vi "Test Lift Core.vi"(8 "Speed":dbl, 11 "Target Height":dbl) -> ()   [LabVIEW 2014]
uses:
  Begin/Global RefNums.vi
  Begin/Global Variables.vi
  <vilib>/addons/control/pid/pid.llb/PID (DBL).vi
  <vilib>/addons/control/pid/NI_PID_pid.lvlib
panel:
  in  "Clear Graph":bool
  out "Graph":cluster{"X":dbl, "Y":dbl}[](graph)
  in  "Speed Offset":dbl
  in  "Right PID gains":T1={"proportional gain (Kc)"=0.002, "integral time (Ti, min)"=0.0, "derivative time (Td, min)"=0.0005} {"derivative time (Td, min)" format="%.7f"; "integral time (Ti, min)" format="%.7f"; "proportional gain (Kc)" format="%.7f"}
  in  "Left PID gains":T1={"proportional gain (Kc)"=0.002, "integral time (Ti, min)"=0.0, "derivative time (Td, min)"=0.0005} {"derivative time (Td, min)" format="%.7f"; "integral time (Ti, min)" format="%.7f"; "proportional gain (Kc)" format="%.7f"}
  in  "Velocity gains":T1={"proportional gain (Kc)"=0.002, "integral time (Ti, min)"=0.0, "derivative time (Td, min)"=0.0} {"derivative time (Td, min)" format="%.7f"; "integral time (Ti, min)" format="%.7f"; "proportional gain (Kc)" format="%.7f"}
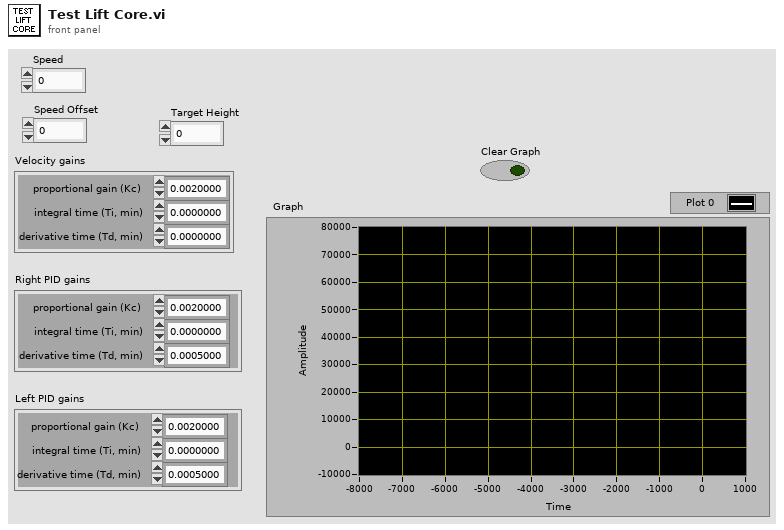
[diagram p1: front panel]
types:
  T1 = cluster{"proportional gain (Kc)":dbl, "integral time (Ti, min)":dbl, "derivative time (Td, min)":dbl}
  T2 = typedef "WPI_EncoderDevRef.ctl" = cluster{"DevStatus":errorcluster, "EncoderIndex":T3, "CounterIndex":T4, "DistancePerCount":dbl, "Decoding Type":T5}
  T3 = typedef "FPGA_EncoderIdx.ctl" = enum8{"Enc 0", "Enc 1", "Enc 2", "Enc 3", "Enc 4", "Enc 5", "Enc 6", "Enc 7", "Invalid"}
  T4 = typedef "FPGA_CounterCtrSystemIndex.ctl" = enum8{"Ctr 0", "Ctr 1", "Ctr 2", "Ctr 3", "Ctr 4", "Ctr 5", "Ctr 6", "Ctr 7", "Invalid"}
  T5 = typedef "WPI_EncoderType.ctl" = enum16{"1x", "2x", "4x"}
  T6 = typedef "WPI_MotorControlDeviceRef.ctl" = cluster{"DeviceStatus":errorcluster, "Type":T7, "PWM":cluster{"Controller":T8, "PWM Channel":T9, "DeadBand":T10}, "CAN":cluster{"Device Number":u8, "Control Mode":T11, "Semaphore":T12, "Max Vout":dbl, "TalonSRX Control Mode":T13}, "Invert":bool, "TransformRef":T14, "InvTransformRef":T14}
  T7 = typedef "WPI_MotorControlType.ctl" = enum16{"PWM", "CAN", "CANTalonSRX"}
  T8 = typedef "FPGA_TypedefDigitalModule.ctl" = enum16{"Controller 1"}
  T9 = typedef "FPGA_DIOPWMChannel.ctl" = enum8{"PWM 0", "PWM 1", "PWM 2", "PWM 3", "PWM 4", "PWM 5", "PWM 6", "PWM 7", "PWM 8", "PWM 9", "PWM MXP 0", "PWM MXP 1", "PWM MXP 2", "PWM MXP 3", "PWM MXP 4", "PWM MXP 5", "PWM MXP 6", "PWM MXP 7", "PWM MXP 8", "PWM MXP 9", "Invalid"}
  T10 = typedef "WPI_PWMDeadband.ctl" = cluster{"Name":string, "maxPositivePwm":i32, "minPositivePwm":i32, "centerPwm":i32, "maxNegativePwm":i32, "minNegativePwm":i32, "angularRange":u16}
  T11 = typedef "WPI_CANJaguar_ControlMode.ctl" = enum8{"Percent VBus", "Current", "Speed", "Position", "Voltage"}
  T12 = typedef "Semaphore RefNum" = refnum<k1>
  T13 = typedef "WPI_CANTalonSRX_APIControlMode.ctl" = enum8{"Percent VBus", "Speed", "Position", "Slave", "Unchanged / Invalid"}
  T14 = typedef "WPI_PWMTransform_ConPane.ctl" = refnum<vi>
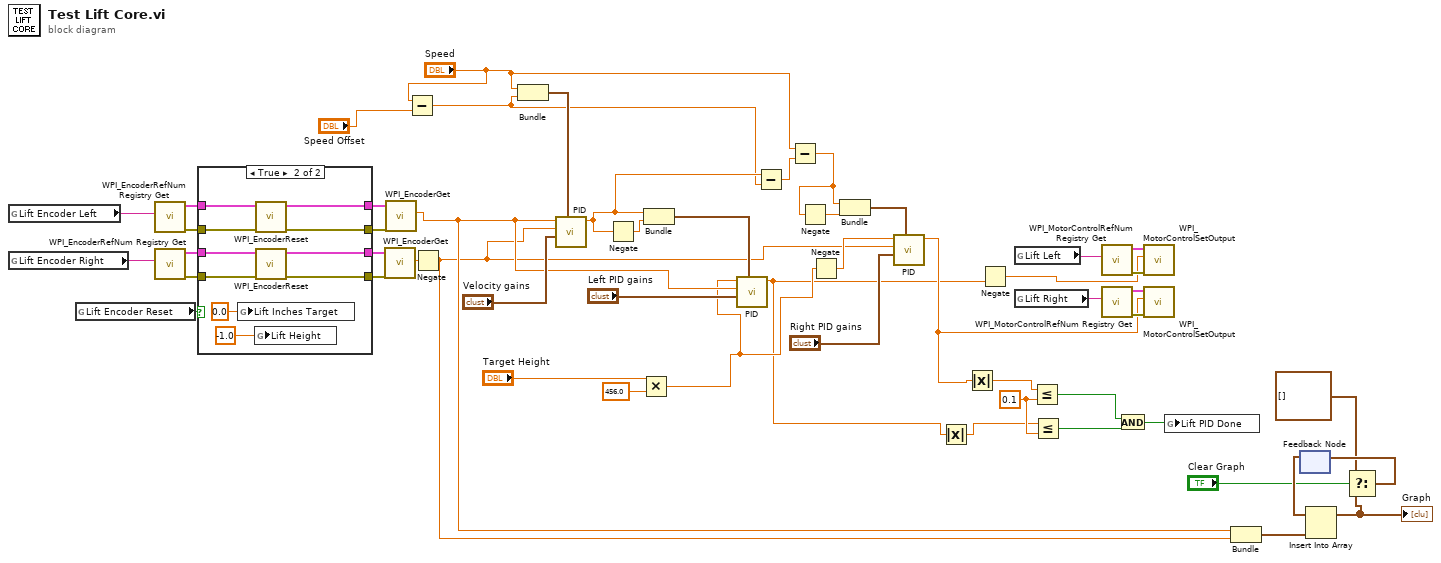
[diagram p0: block diagram]
diagram:
  w26 = 0.1 ("y")
  n1 = global read "Global RefNums.vi" "Lift Encoder Left"() -> (w39:string)
  n2 = global read "Global RefNums.vi" "Lift Encoder Right"() -> (w38:string)
  n3 = global read "Global Variables.vi" "Lift Encoder Reset"() -> (w37:bool)
  n4 = call <vilib>:"WPI_EncoderRefNum Registry Get.vi"("refnum name"=w39) -> ("error out"=w43:errorcluster, "EncoderDevRef"=w42:T2)  [unwired: 9 in]
  n5 = call <vilib>:"WPI_EncoderRefNum Registry Get.vi"("refnum name"=w38) -> ("error out"=w40:errorcluster, "EncoderDevRef"=w41:T2)  [unwired: 9 in]
  n6 = case shown="True" w37 {
    tunnel: w40 -> [w54 w67]
    tunnel: w41 -> [w55 w66]
    tunnel: w43 -> [w56 w64]
    tunnel: w42 -> [w57 w65]
    tunnel: [w57 w63] -> w44
    tunnel: [w55 w62] -> w45
    tunnel: [w54 w61] -> w46
    tunnel: [w56 w60] -> w47
    frame False {
    }
    frame True {
      n7 = global write "Global Variables.vi" "Lift Inches Target"(0.0 ("Lift Inches Target")) -> ()
      n8 = global write "Global Variables.vi" "Lift Height"(-1.0 ("Lift Inches Target")) -> ()
      n9 = call <vilib>:"WPI_EncoderReset.vi"("error in (no error)"=w64, "EncoderDevRef"=w65) -> ("error out"=w60:errorcluster, "EncoderDevRef"=w63:T2)  [unwired: 8 in]
      n10 = call <vilib>:"WPI_EncoderReset.vi"("error in (no error)"=w67, "EncoderDevRef"=w66) -> ("error out"=w61:errorcluster, "EncoderDevRef"=w62:T2)  [unwired: 8 in]
    }
  }
  n11 = call <vilib>:"WPI_EncoderGet.vi"("error in (no error)"=w46, "EncoderDevRef"=w45) -> ("Distance"=w8:dbl)  [unwired: 4 in, 5 out]
  n12 = call <vilib>:"WPI_EncoderGet.vi"("error in (no error)"=w47, "EncoderDevRef"=w44) -> ("Distance"=w11:dbl)  [unwired: 4 in, 5 out]
  n13 = Subtract(x="Speed", y="Speed Offset") -> (x-y=w17:dbl)
  n14 = Negate(x=w8) -> (-x=w7:dbl)
  n15 = Bundle("Speed"="Speed", w17) -> (w24:cluster{"Speed":dbl, dbl})  [unwired: 1 in]
  n16 = call-poly <vilib>:"PID.vi"("output range"=w24, "PID gains"="Velocity gains", "process variable"=w7, "setpoint"=w11) -> ("output"=w33:dbl)  [unwired: 6 in, 1 out]
  n17 = Negate(x=w33) -> (-x=w30:dbl)
  n18 = Multiply(x="Target Height", y=456.0) -> (x*y=w10:dbl)
  n19 = Bundle("output"=w33, w30) -> (w36:cluster{"output":dbl, dbl})  [unwired: 1 in]
  n20 = call-poly <vilib>:"PID.vi"("output range"=w36, "PID gains"="Left PID gains", "process variable"=w11, "setpoint"=w10) -> ("output"=w4:dbl)  [unwired: 6 in, 1 out]
  n21 = Subtract(x=w33, y=w17) -> (x-y=w34:dbl)
  n22 = Subtract(x="Speed", y=w34) -> (x-y=w1:dbl)
  n23 = Negate(x=w1) -> (-x=w2:dbl)
  n24 = Negate(x=w10) -> (-x=w9:dbl)
  n25 = Bundle(w1, w2) -> (w29:cluster{dbl, dbl})  [unwired: 1 in]
  n26 = call-poly <vilib>:"PID.vi"("output range"=w29, "PID gains"="Right PID gains", "process variable"=w7, "setpoint"=w9) -> ("output"=w5:dbl)  [unwired: 6 in, 1 out]
  n27 = Absolute Value(x=w4) -> (abs(x)=w3:dbl)
  n28 = Absolute Value(x=w5) -> (abs(x)=w6:dbl)
  n29 = Negate(x=w4) -> (-x=w12:dbl)
  n30 = global read "Global RefNums.vi" "Lift Left"() -> (w49:string)
  n31 = global read "Global RefNums.vi" "Lift Right"() -> (w48:string)
  n32 = Less Or Equal?(x=w6, y=w26) -> (x <= y?=w28:bool)
  n33 = Less Or Equal?(x=w3, y=w26) -> (x <= y?=w27:bool)
  n34 = call <vilib>:"WPI_MotorControlRefNum Registry Get.vi"("refnum name"=w49) -> ("error out"=w53:errorcluster, "MotorControlDevRef"=w52:T6)  [unwired: 9 in]
  n35 = call <vilib>:"WPI_MotorControlRefNum Registry Get.vi"("refnum name"=w48) -> ("error out"=w50:errorcluster, "MotorControlDevRef"=w51:T6)  [unwired: 9 in]
  n36 = And(x=w28, y=w27) -> (x .and. y?=w25:bool)
  n37 = call <vilib>:"WPI_MotorControlSetOutput.vi"("error in (no error)"=w53, "Output"=w12, "MotorControlDevRef"=w52) -> ()  [unwired: 6 in, 3 out]
  n38 = call <vilib>:"WPI_MotorControlSetOutput.vi"("error in (no error)"=w50, "Output"=w5, "MotorControlDevRef"=w51) -> ()  [unwired: 6 in, 3 out]
  n39 = global write "Global Variables.vi" "Lift PID Done"(w25) -> ()
  n40 = Bundle("Distance"=w11, w7) -> (w23:cluster{"Distance":dbl, dbl})  [unwired: 1 in]
  n41 = feedback #1() -> (w22:cluster{"Distance":dbl, "Distance":dbl}[])  [unwired: 1 in]
  n42 = Insert Into Array(array=w22, new element=w23) -> (w21:cluster{"Distance":dbl, "Distance":dbl}[])  [unwired: 1 in]
  "Graph" <- w21
  n43 = Select(t=cluster{"Distance":dbl, "Distance":dbl}[] [], s="Clear Graph", f=w21) -> (s? t:f=w20:cluster{"Distance":dbl, "Distance":dbl}[])
  n44 = feedback-in #1(w20) -> ()
